vi "Save as Text2.vi"(7 "action":string="Save", 8 "error in":errorcluster, 10 "file path (use dialog)":path, 11 "data in":sgl[](array[numeric])) -> (0 "error out":errorcluster)   [LabVIEW 2018]
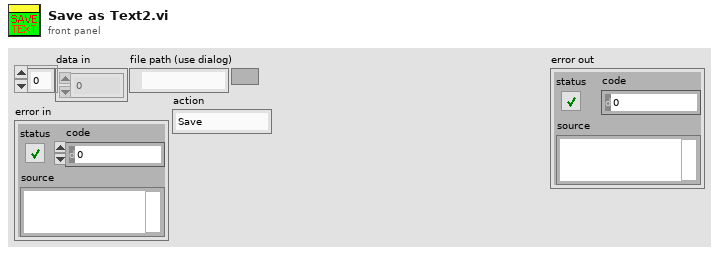
[diagram p1: front panel]
types:
  T1 = enum16{"open", "replace", "create", "open or create", "replace or create", "replace or create with confirmation"}
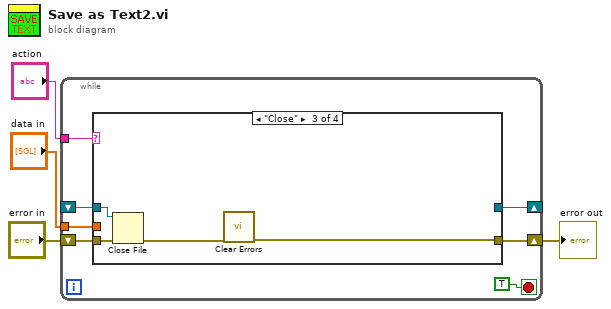
[diagram p0: block diagram]
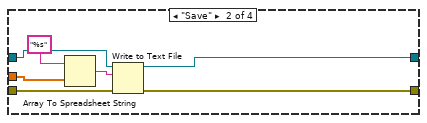
[diagram p3: hidden frame]
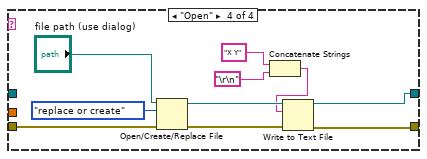
[diagram p4: hidden frame]
diagram:
  n1 = while {
    tunnel: "action" -> [w10]
    tunnel: "data in" -> [w9]
    shift-right: [w7] -> w2
    shift-left: "error in" -> [w8]
    shift-right: [w6] -> _
    shift-left: _ -> [w5]
    stop <- TRUE stop-if-true
    n2 = case shown="\"Close\"" w10 {
      tunnel: w9 -> [_ w16 _ _]
      tunnel: w8 -> [w13 w18 w24 w34]
      tunnel: [w13 w20 w21 w30] -> w7
      tunnel: [w12 w19 _ w29] -> w6
      tunnel: w5 -> [w12 w17 w23 _]
      frame "False", Default {
      }
      frame "Save" {
        n3 = Array To Spreadsheet String(array=w16, 3:"%s" ("format string")) -> (spreadsheet string=w15:string)  [unwired: 1 in]
        n4 = Write to Text File(file (use dialog)=w17, text=w15, error in=w18) -> (refnum out=w19:refnum<file>, error out=w20:errorcluster)  [unwired: 1 in, 1 out]
      }
      frame "Close" {
        n5 = Close File(refnum=w23, error in=w24) -> (error out=w22:errorcluster)  [unwired: 1 out]
        n6 = call <vilib>:"Clear Errors.vi"("error in (no error)"=w22) -> ("error out"=w21:errorcluster)  [unwired: 5 in, 1 out]
      }
      frame "Open" {
        n7 = Open/Create/Replace File(file path (use dialog)="file path (use dialog)", error in=w34, operation (0:open)=T1."replace or create") -> (refnum out=w28:refnum<file>, error out=w31:errorcluster)  [unwired: 3 in, 1 out]
        n8 = Concatenate Strings("X Y" ("text"), "\r\n") -> (w25:string)
        n9 = Write to Text File(file (use dialog)=w28, text=w25, error in=w31) -> (refnum out=w29:refnum<file>, error out=w30:errorcluster)  [unwired: 1 in, 1 out]
      }
    }
  }
  "error out" <- w2
